vi "Cycle.vi"(8 "error in (no error)":errorcluster, 11 "EyeCalibration In":refnum<class "EyeCalibration.lvclass">) -> (0 "error out":errorcluster, 3 "EyeCalibration Out":refnum<class "EyeCalibration.lvclass">)   [LabVIEW 2010, in "EyeCalibration.lvclass"]
uses:
  EyeCalibration.lvclass
  MatlabExperiment/MatlabExperiment.lvclass
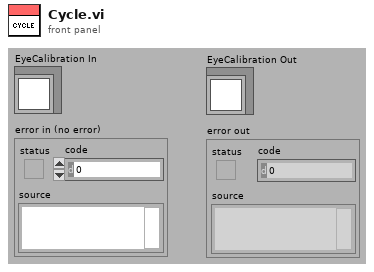
[diagram p1: front panel]
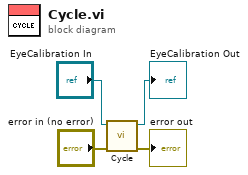
[diagram p0: block diagram]
diagram:
  n1 = call-parent "Cycle.vi"("error in (no error)"="error in (no error)", "MatlabExperiment In"="EyeCalibration In") -> ("error out"=→"error out":errorcluster, "MatlabExperiment Out"=→"EyeCalibration Out":refnum<class "EyeCalibration.lvclass">)  [unwired: 8 in]
